vi "BinaryOffset.vi"(10 "Offset in":bool[](array[boolean]), 11 "Number in":bool[](array[boolean])) -> (3 "Array out":bool[](array[boolean]))   [LabVIEW 2021]
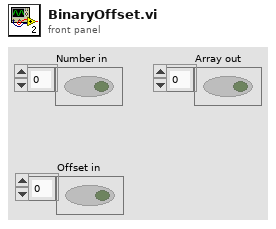
[diagram p1: front panel]
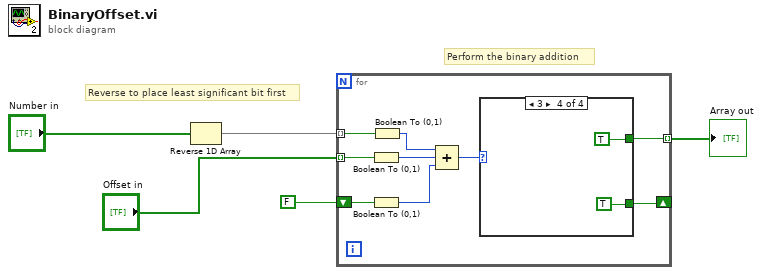
[diagram p0: block diagram]
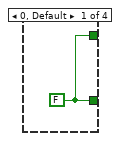
[diagram p2: hidden frame]
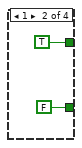
[diagram p3: hidden frame]
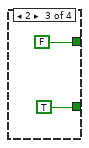
[diagram p4: hidden frame]
diagram:
  # "Perform the binary addition"
  # "Reverse to place least significant bit first"
  n1 = Reverse 1D Array(array="Number in") -> (reversed array=w4:bool[])
  n2 = for {
    tunnel: w4 -> [w14] mode=indexing
    tunnel: "Offset in" -> [w13] mode=indexing
    shift-right: [w7] -> _
    shift-left: FALSE -> [w12]
    tunnel: [w6] -> w1 mode=indexing
    n3 = Boolean To (0,1)(Boolean=w13) -> (0, 1=w10:i16)
    n4 = Boolean To (0,1)(Boolean=w12) -> (0, 1=w9:i16)
    n5 = Boolean To (0,1)(Boolean=w14) -> (0, 1=w11:i16)
    n6 = Compound Arithmetic op=ADD(w11, w10, w9) -> (w8:i16)
    n7 = case shown="3" w8 {
      tunnel: [w15 FALSE TRUE TRUE] -> w7
      tunnel: [w15 TRUE FALSE TRUE] -> w6
      frame 0, Default {
        w15 = FALSE
      }
      frame 1 {
      }
      frame 2 {
      }
      frame 3 {
      }
    }
  }
  "Array out" <- w1
